vi "encodeUInt.vi"(8 "error in (no error)":errorcluster, 10 "Variant":variant) -> (0 "error out":errorcluster, 2 "Array":u8[](array[numeric]) format="%.0x")   [LabVIEW 2016, in "MsgPack.lvlib"]
uses:
  MsgPack.lvlib
  <vilib>/Utility/Data Type/NI_Data Type.lvlib
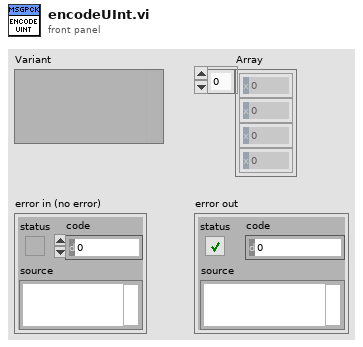
[diagram p1: front panel]
types:
  T1 = typedef "NI_Data Type.lvlib/Data Type.ctl" = enum8{"Invalid Type", "Void", "I8", "I16", "I32", "I64", "U8", "U16", "U32", "U64", "Single Float", "Double Float", "Extended Float", "Single Complex", "Double Complex", "Extended Complex", "Enum U8", "Enum U16", "Enum U32", "Enum U64", "Single Float With Unit", "Double Float With Unit", "Extended Float With Unit", "Single Complex with Unit", "Double Complex with Unit", "Extended Complex with Unit", "Boolean", "String", "Path", "Picture", "Tag", "Array", "Cluster", "Variant", "LV Variant", "Waveform", "Timestamp", "Digital Waveform", "Digital Data", "ExpressData", "Refnum", "External Data", "VI", "Poly VI", "LabVIEW Class Instance", "Fixed Point"}
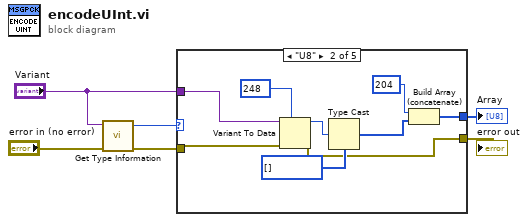
[diagram p0: block diagram]
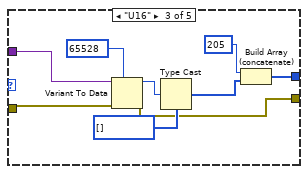
[diagram p3: hidden frame]
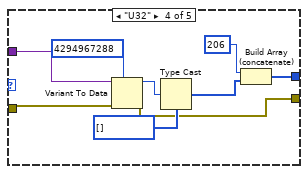
[diagram p4: hidden frame]
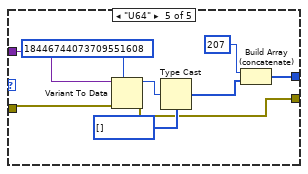
[diagram p5: hidden frame]
diagram:
  n1 = call <vilib>:"Get Type Information.vi"("error in (no error)"="error in (no error)", "Variant"="Variant") -> ("error out"=w5:errorcluster, "Type"=w6:T1)  [unwired: 5 in, 3 out]
  n2 = case shown="\"U8\"" w6 {
    tunnel: w5 -> [w7 w16 w25 w34 w43]
    tunnel: "Variant" -> [_ w15 w24 w33 w42]
    tunnel: [_ w9 w18 w27 w36] -> w3
    tunnel: [w7 w8 w17 w26 w35] -> w2
    frame "Invalid Type", Default {
    }
    frame "U8" {
      n3 = Variant To Data(error in=w16, type=u8 248, Variant=w15) -> (data=w12:u8, error out=w8:errorcluster)
      n4 = Type Cast(type=u8[] [], x=w12) -> (*(type *) &x=w10:u8[])
      n5 = Build Array (concatenate)(u8 204, w10) -> (w9:u8[])
    }
    frame "U16" {
      n6 = Variant To Data(error in=w25, type=u16 65528, Variant=w24) -> (data=w21:u16, error out=w17:errorcluster)
      n7 = Type Cast(type=u8[] [], x=w21) -> (*(type *) &x=w19:u8[])
      n8 = Build Array (concatenate)(u8 205, w19) -> (w18:u8[])
    }
    frame "U32" {
      n9 = Variant To Data(error in=w34, type=u32 4294967288, Variant=w33) -> (data=w30:u32, error out=w26:errorcluster)
      n10 = Type Cast(type=u8[] [], x=w30) -> (*(type *) &x=w28:u8[])
      n11 = Build Array (concatenate)(u8 206, w28) -> (w27:u8[])
    }
    frame "U64" {
      n12 = Variant To Data(error in=w43, type=u64 18446744073709551608, Variant=w42) -> (data=w39:u64, error out=w35:errorcluster)
      n13 = Type Cast(type=u8[] [], x=w39) -> (*(type *) &x=w37:u8[])
      n14 = Build Array (concatenate)(u8 207, w37) -> (w36:u8[])
    }
  }
  "Array" <- w3
  "error out" <- w2
